vi "Generate Signal.vi"() -> (4 "AI N-1":i16, 6 "AI N":i16)   [LabVIEW 2014]
doc: "This VI generates two samples every iteration from a waveform of a 3MHz sine tone sampled at 200MHz. This VI is intended to be run in a 100MHz clock domain inside of a Single Cycle Timed Loop."
uses:
  <vilib>/rvi/DataTransferAndStorage/Container/Common/niFpgaContainerGetUniqueNameForEmu.vi
  <vilib>/rvi/DataTransferAndStorage/Container/Common/niFpgaContainerSetEmuInfo.vi
  <vilib>/rvi/eio/common/nirviEmuReportErrorAndStop.vi
  <vilib>/rvi/DataTransferAndStorage/Container/Common/niFpgaContainerExecOnDevCompGetState.vi
  <vilib>/rvi/Emulation/niFpgaEmulationIsFPGAContextNoSignature.vi
  <vilib>/rvi/Emulation/niFpgaProcessEmulError.vi
  <vilib>/rvi/Emulation/niFpgaSctlEmulationGetInTimedLoop.vi
  <vilib>/rvi/errors/nirviReportUnexpectedCaseInternalError (U32).vi
  <vilib>/rvi/Memory/Memory_Emulation/niFpgaMemoryEmulationCacheClearOnFirstRun.vi
  <vilib>/rvi/Memory/Memory_Emulation/nirvimemoryEmulationManagerCache_MakeExclusive.vi
  <vilib>/rvi/Memory/Memory_Emulation/niFpgaMemoryEmulationValidateCache.vi
  <vilib>/rvi/Memory/Memory_Emulation/nirvimemoryEmulationManagerCache_InsertValue.vi
  <vilib>/Utility/error.llb/Clear Errors.vi
  <vilib>/rvi/Memory/Memory_Emulation/nirvimemoryEmulationManagerCache_ReleaseExclusive.vi
  <vilib>/rvi/Memory/Memory_Emulation/nirvimemoryEmulationManagerCache_GetValue.vi
  <vilib>/rvi/Memory/Memory_Emulation/nirvimemoryEmulationManagerCache_SetValue.vi
  <vilib>/rvi/Emulation/niFpgaSctlEmulationResourceMgr.vi
  <vilib>/rvi/LocalResourceManager/LocalResourceManager.xnode
  <vilib>/rvi/DataTransferAndStorage/Container/XNode/niFpgaContainer.xnode
  <vilib>/rvi/Memory/Memory_Emulation/niFpgaMemoryEmulationRefIn.vi
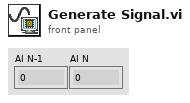
[diagram p1: front panel]
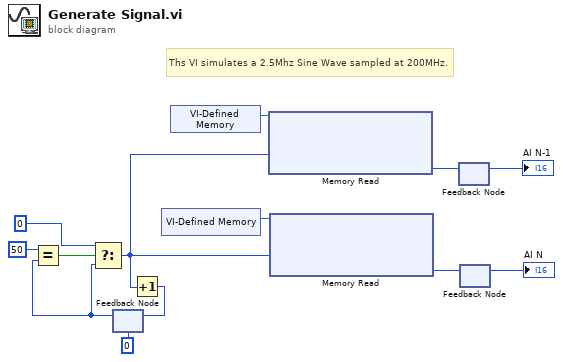
[diagram p0: block diagram]
diagram:
  # "Ths VI simulates a 2.5Mhz Sine Wave sampled at 200MHz."
  n1 = feedback #1(u32 0 ("Address")) -> (w5:u32)
  n2 = Equal?(x=u32 50, y=w5) -> (x = y?=w8:bool)
  n3 = Select(t=u32 0 ("Address"), s=w8, f=w5) -> (s? t:f=w7:u32)
  n4 = Increment(x=w7) -> (x+1=w6:u32)
  n5 = feedback-in #1(w6) -> ()
  n6 = xnode "VI-Defined Memory"() -> ("Memory Out"=w12:refnum<k21>)
  n7 = xnode "VI-Defined Memory"() -> ("Memory Out"=w13:refnum<k21>)
  n8 = xnode ("Memory Read")("Address"=w7, "Memory In"=w13) -> ("Data"=w4:i16)  [unwired: 1 out]
  n9 = xnode ("Memory Read")("Address"=w7, "Memory In"=w12) -> ("Data"=w3:i16)  [unwired: 1 out]
  n10 = feedback-in #2(w4) -> ()
  n11 = feedback #2() -> (→"AI N-1":i16)  [unwired: 1 in]
  n12 = feedback #3() -> (→"AI N":i16)  [unwired: 1 in]
  n13 = feedback-in #3(w3) -> ()
